vi "Read Attenuator.vi"(11 "Spectrum Analyzer in":refnum<class "Spectrum Analyzer.lvclass">) -> (2 "Attenuator":dbl, 3 "Spectrum Analyzer out":refnum<class "Spectrum Analyzer.lvclass">)   [LabVIEW 2020, in "Spectrum Analyzer.lvclass"]
uses:
  Spectrum Analyzer.lvclass
  Spectrum Analyzer.lvclass/Spectrum Analyzer.ctl
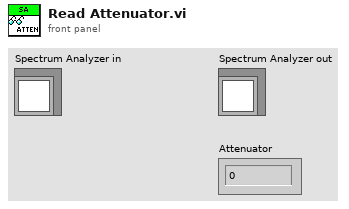
[diagram p1: front panel]
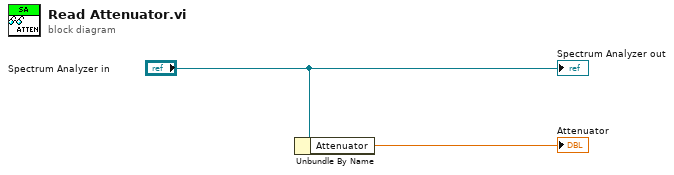
[diagram p0: block diagram]
diagram:
  n1 = Unbundle By Name("Spectrum Analyzer in") -> ("Attenuator"=→"Attenuator":dbl)
  "Spectrum Analyzer out" <- "Spectrum Analyzer in"
